vi "Translation3d_GetDistance.vi"(9 "other Translation":T1 {"Z" format="%14.3f"; "Y" format="%14.3f"; "X" format="%14.3f"}, 11 "In Translation":T1 {"Z" format="%14.3f"; "Y" format="%14.3f"; "X" format="%14.3f"}) -> (2 "Distance":dbl)   [LabVIEW 2019, in "Trajectory_Library.lvlib"]
doc: "Calculates the distance between two translations in 2d space.\n\nThis function uses the pythagorean theorem to calculate the distance. distance = sqrt((x2 - x1)^2 + (y2 - y1)^2)\n\nParameters: \n - IN TRANSLATION - This TRANSLATION data structure\n - OTHER TRANSLATION - The translation to compute the distance to.\n\nReturns:\n - Distance - The distance between the two translations."
uses:
  Trajectory_Library.lvlib
  TRANSLATION3D.ctl
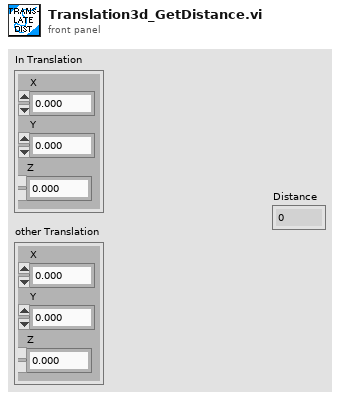
[diagram p1: front panel]
types:
  T1 = typedef "Trajectory_Library.lvlib/TRANSLATION3D.ctl" = cluster{"X":dbl, "Y":dbl, "Z":dbl}
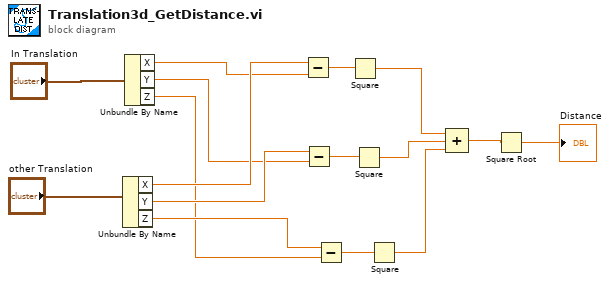
[diagram p0: block diagram]
diagram:
  n1 = Unbundle By Name("other Translation") -> ("X"=w14:dbl, "Y"=w12:dbl, "Z"=w10:dbl)
  n2 = Unbundle By Name("In Translation") -> ("X"=w13:dbl, "Y"=w11:dbl, "Z"=w9:dbl)
  n3 = Subtract(x=w14, y=w13) -> (x-y=w5:dbl)
  n4 = Subtract(x=w12, y=w11) -> (x-y=w6:dbl)
  n5 = Subtract(x=w10, y=w9) -> (x-y=w4:dbl)
  n6 = Square(x=w5) -> (x^2=w8:dbl)
  n7 = Square(x=w6) -> (x^2=w7:dbl)
  n8 = Square(x=w4) -> (x^2=w3:dbl)
  n9 = Compound Arithmetic op=ADD(w8, w7, w3) -> (w2:dbl)
  n10 = Square Root(x=w2) -> (sqrt(x)=→"Distance":dbl)
